vi "LDAP Authentication.vi"(8 "error in (no error)":errorcluster, 9 "Password":string, 10 "User Name":string, 11 "Server":string) -> (0 "error out":errorcluster, 3 "Valid?":bool)   [LabVIEW 2016, in "LDAP Authentication.lvclass"]
uses:
  LDAP Authentication/LDAP Authentication.lvclass
  System.DirectoryServices.AccountManagement
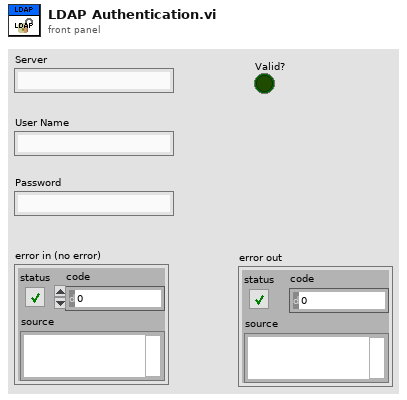
[diagram p1: front panel]
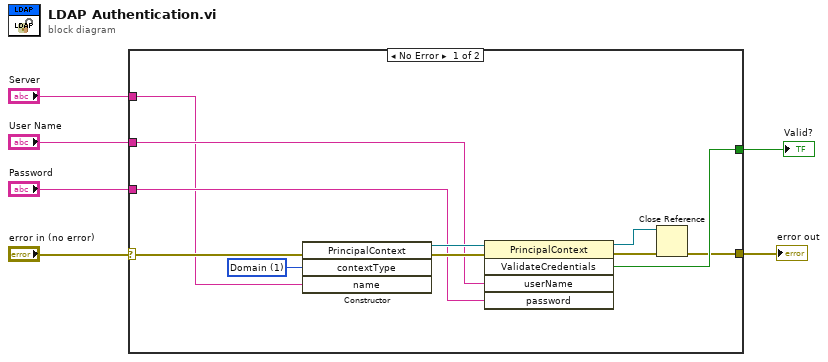
[diagram p0: block diagram]
diagram:
  n1 = case shown="No Error" "error in (no error)" {
    selector: "error in (no error)" -> [w8 w18]
    tunnel: "User Name" -> [w12 _]
    tunnel: [w11 _] -> w5
    tunnel: [w10 w18] -> w4
    tunnel: "Password" -> [w9 _]
    tunnel: "Server" -> [w7 _]
    frame No Error {
      w17 = 1 items=["Machine", "Domain", "ApplicationDirectory"] ("contextType")
      n2 = constructor class="PrincipalContext"(error in=w8, "contextType"=w17, "name"=w7) -> (reference out=w16:refnum<k24>, error out=w15:errorcluster)  [unwired: 2 in, 3 out]
      n3 = invoke class="PrincipalContext" method="ValidateCredentials"(reference=w16, error in=w15, "userName"=w12, "password"=w9) -> (reference out=w14:refnum<k24>, error out=w13:errorcluster, "ValidateCredentials"=w11:bool)  [unwired: 1 in, 2 out]
      n4 = Close Reference(reference=w14, error in (no error)=w13) -> (error out=w10:errorcluster)
    }
    frame Error {
    }
  }
  "Valid?" <- w5
  "error out" <- w4
